vi "FTW-Reflection-Array.vi"(7 "Array":variant) -> (8 "Default Array Element":variant, 10 "Number of Dimensions":i32)   [LabVIEW 2014]
panel:
  # "Inputs"
  # "Outputs"
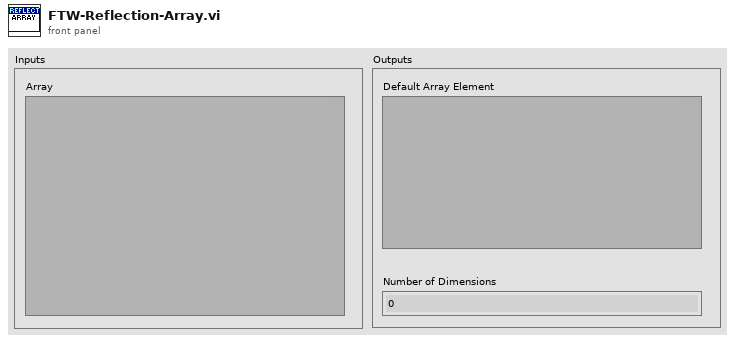
[diagram p1: front panel]
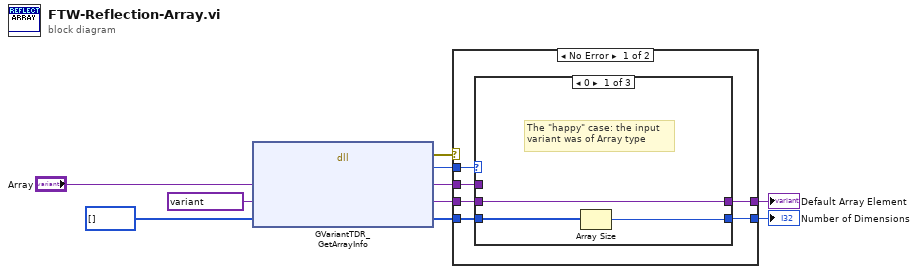
[diagram p0: block diagram]
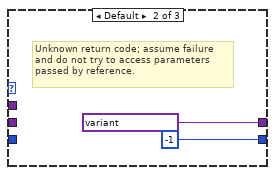
[diagram p2: hidden frame]
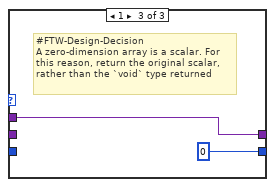
[diagram p3: hidden frame]
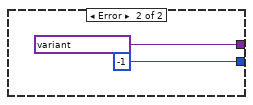
[diagram p4: hidden frame]
diagram:
  n1 = dll-call lib="LabVIEW" fn="GVariantTDR_GetArrayInfo"("Array as a Variant"="Array", "Default Array Element"=variant, "Dimensions"=i32[] []) -> (error out=w2:errorcluster, "Return Value"=w1:i32, "Array as a Variant"=w3:variant, "Default Array Element"=w4:variant, "Dimensions"=w7:i32[])  [unwired: 3 in, 1 out]
  n2 = case shown="No Error" w2 {
    tunnel: [w12 -1] -> w10
    tunnel: w7 -> [w16 _]
    tunnel: [w13 variant] -> w5
    tunnel: w4 -> [w14 _]
    tunnel: w3 -> [w15 _]
    tunnel: w1 -> [w11 _]
    frame No Error {
      n3 = case shown="0" w11 {
        tunnel: w16 -> [w18 _ _]
        tunnel: w15 -> [_ _ w23]
        tunnel: w14 -> [w19 _ _]
        tunnel: [w19 variant w23] -> w13
        tunnel: [w17 -1 0] -> w12
        frame 0 {
          # "The \"happy\" case: the input\nvariant was of Array type"
          n4 = Array Size(array=w18) -> (size(s)=w17:i32)
        }
        frame Default {
          # "Unknown return code; assume failure\nand do not try to access parameters\npassed by reference."
        }
        frame 1 {
          # "#FTW-Design-Decision\nA zero-dimension array is a scalar. For\nthis reason, return the original scalar,\nrather than the `void` type returned"
        }
      }
    }
    frame Error {
    }
  }
  "Default Array Element" <- w5
  "Number of Dimensions" <- w10
